vi "emi_FP Hide.vi"(5 "VI Refnum(This vi)":refnum<vi>, 7 "Show time s(0)":dbl, 9 "error in (no error)":errorcluster) -> (6 "VI Refnum":refnum<vi>, 10 "error out":errorcluster)   [LabVIEW 2011]
doc: "Fades VI from current transparensy to \"Transparansy %(100)\". \nUses time instead of number of iterations to avoid overly long fade ins when processing power is at a premium.\ns\nIf no VI ref in, then the VI containing this VI is used.\nIf VI has multiple panes, only the first pane will be used.\n\nOn error in: Tries to run like normal (Does not run.removed 110126)"
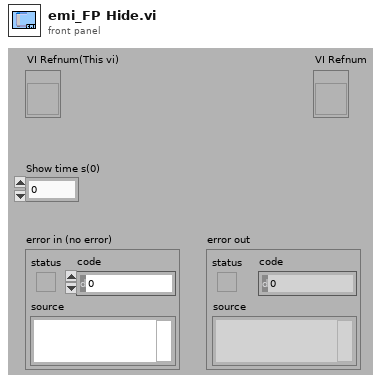
[diagram p1: front panel]
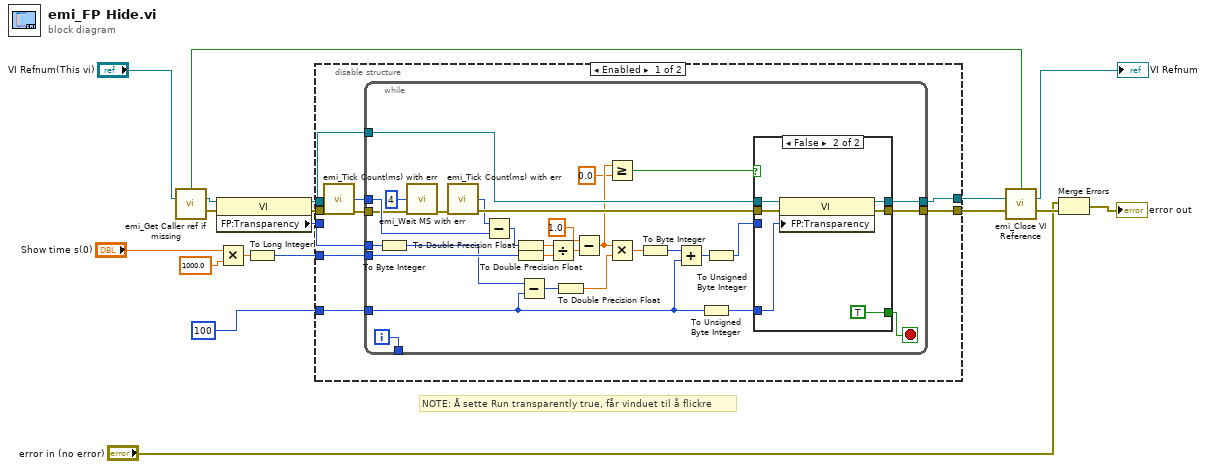
[diagram p0: block diagram]
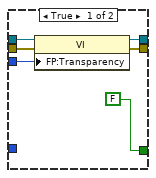
[diagram p2: hidden frame]
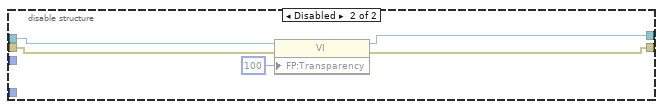
[diagram p3: hidden frame]
diagram:
  # "NOTE: Å sette Run transparently true, får vinduet til å flickre"
  n1 = call "emi_Get Caller ref if missing.vi"("VI Refnum(Calling VI)"="VI Refnum(This vi)") -> ("Ref Generated"=w14:bool, "VI Refnum Out"=w5:refnum<vi>, "error out"=w13:errorcluster)  [unwired: 12 in]
  n2 = property class="VI"(reference=w5, error in=w13) -> (reference out=w11:refnum<vi>, error out=w12:errorcluster, "FP:Transparency"=w10:u8)
  n3 = Multiply(x="Show time s(0)", y=1000.0) -> (x*y=w8:dbl)
  n4 = To Long Integer(number=w8) -> (32bit integer=w7:i32)
  n5 = disable-structure shown="Enabled" {
    disable-tunnel: w12 -> [w27 w74]
    disable-tunnel: w11 -> [w25 w72]
    disable-tunnel: w10 -> [w23 _]
    disable-tunnel: w7 -> [w22 _]
    disable-tunnel: [w21 w70] -> w6
    disable-tunnel: i8 100 ("Target Transparensy %(100)") -> [w20 _]
    disable-tunnel: [w19 w71] -> w3
    frame Enabled {
      n6 = call "emi_Tick Count(ms) with err.vi"("error in (no error)"=w27) -> ("millisecond timer value"=w24:u32, "error out"=w26:errorcluster)  [unwired: 13 in]
      n7 = while {
        tunnel: w26 -> [w51]
        tunnel: w25 -> [w55]
        tunnel: w24 -> [w52]
        tunnel: [w57] -> w21
        tunnel: [w54] -> w19
        tunnel: w23 -> [w35]
        tunnel: w22 -> [w47]
        tunnel: [w39] -> _
        tunnel: w20 -> [w28]
        i -> [w39]
        stop <- w40 stop-if-true
        n8 = To Byte Integer(number=w35) -> (8bit integer=w34:i8)
        n9 = call "emi_Wait MS with err.vi"("milliseconds to wait(0)"=u32 4, "error in (no error)"=w51) -> ("error out"=w50:errorcluster)  [unwired: 13 in]
        n10 = call "emi_Tick Count(ms) with err.vi"("error in (no error)"=w50) -> ("millisecond timer value"=w53:u32, "error out"=w56:errorcluster)  [unwired: 13 in]
        n11 = Subtract(x=w53, y=w52) -> (x-y=w48:u32)
        n12 = To Double Precision Float(number=w48) -> (double precision float=w46:dbl)
        n13 = To Double Precision Float(number=w47) -> (double precision float=w45:dbl)
        n14 = Subtract(x=w34, y=w28) -> (x-y=w36:i8)
        n15 = Divide(x=w46, y=w45) -> (x/y=w44:dbl)
        n16 = To Double Precision Float(number=w36) -> (double precision float=w38:dbl)
        n17 = Subtract(x=1.0, y=w44) -> (x-y=w31:dbl)
        n18 = Greater Or Equal?(x=w31, y=0.0) -> (x >= y?=w29:bool)
        n19 = Multiply(x=w31, y=w38) -> (x*y=w41:dbl)
        n20 = To Byte Integer(number=w41) -> (8bit integer=w42:i8)
        n21 = Add(x=w42, y=w28) -> (x+y=w37:i8)
        n22 = To Unsigned Byte Integer(number=w28) -> (unsigned 8bit integer=w32:u8)
        n23 = To Unsigned Byte Integer(number=w37) -> (unsigned 8bit integer=w33:u8)
        n24 = case shown="False" w29 {
          tunnel: [w63 w66] -> w57
          tunnel: w56 -> [w62 w68]
          tunnel: w55 -> [w61 w67]
          tunnel: [w60 w65] -> w54
          tunnel: [FALSE TRUE] -> w40
          tunnel: w32 -> [_ w64]
          tunnel: w33 -> [w58 _]
          frame True {
            n25 = property class="VI"(reference=w61, error in=w62, "FP:Transparency"=w58) -> (reference out=w60:refnum<vi>, error out=w63:errorcluster)
          }
          frame False {
            n26 = property class="VI"(reference=w67, error in=w68, "FP:Transparency"=w64) -> (reference out=w65:refnum<vi>, error out=w66:errorcluster)
          }
        }
      }
    }
    frame Disabled {
      n27 = property class="VI"(reference=w72, error in=w74, "FP:Transparency"=u8 100 ("Front Panel Window:Transparency")) -> (reference out=w71:refnum<vi>, error out=w70:errorcluster)
    }
  }
  n28 = call "emi_Close VI Reference.vi"("Close ref?(T)"=w14, "VI Refnum"=w3, "error in (no error)"=w6) -> ("VI Refnum Out"=→"VI Refnum":refnum<vi>, "error out"=w18:errorcluster)  [unwired: 11 in]
  n29 = Merge Errors("error in (no error)", w18) -> (→"error out":errorcluster)
